vi "Build Path.vi"(5 "Parallel in":refnum<class "Parallel.lvclass">, 6 "Path Builder":refnum<class "IPath Builder.lvclass">, 7 "Linked List ID":string, 8 "error in (no error)":errorcluster, 11 "Linked List Ref":refnum<data-value>) -> (0 "error out":errorcluster, 2 "Paths":path[](array[path]), 3 "Linked List Ref out":refnum<data-value>)   [LabVIEW 2017]
uses:
  37e9a4a8-58a6-4167-85ed-956ace0f3b24.vi
  Path Builder/IPath Builder/IPath Builder.lvclass
  linked-list/Source/Linked List/ILinkedList/ILinked List.lvclass
  Parallel.lvclass
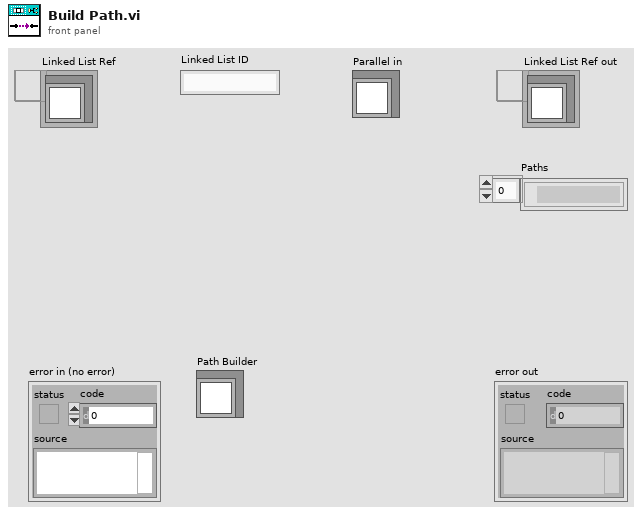
[diagram p1: front panel]
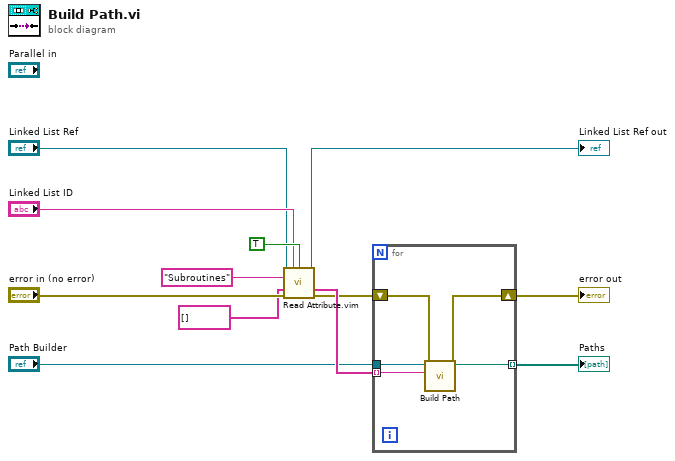
[diagram p0: block diagram]
diagram:
  n1 = call "Read Attribute.vim"("Linked List Ref"="Linked List Ref", "Linked List ID"="Linked List ID", "Include Private?"=TRUE, "Attribute Name"="Subroutines", "Type"=string[] [], "error in (no error)"="error in (no error)") -> ("Linked List Ref out"=→"Linked List Ref out":refnum<data-value>, "Attribute"=w10:string[], "error out"=w9:errorcluster)  [unwired: 4 in, 3 out]
  n2 = for {
    tunnel: w10 -> [w17] mode=indexing
    tunnel: "Path Builder" -> [w14]
    shift-right: [w15] -> w7
    shift-left: w9 -> [w16]
    tunnel: [w13] -> w1 mode=indexing
    n3 = call-dynamic "Build Path.vi"("error in (no error)"=w16, "Path"=w17, "IPath Builder in"=w14) -> ("error out"=w15:errorcluster, "Path"=w13:path)  [unwired: 7 in]
  }
  "error out" <- w7
  "Paths" <- w1
